vi "Obtain Notifier.vi"(7 "Notifier Name":string, 8 "error in":errorcluster, 10 "IMessagePayload.lvclass":refnum<class "IMessagePayload.lvclass">, 11 "NotifierMessageTransport in":refnum<class "NotifierMessageTransport.lvclass">) -> (0 "error out":errorcluster, 3 "NotifierMessageTransport out":refnum<class "NotifierMessageTransport.lvclass">)   [LabVIEW 2016, in "NotifierMessageTransport.lvclass"]
uses:
  NotifierMessageTransport.lvclass
  IMessagePayload/IMessagePayload.lvclass
  NotifierMessageTransport.lvclass/NotifierMessageTransport.ctl
panel:
  # "INPUTS"
  # "OUTPUTS"
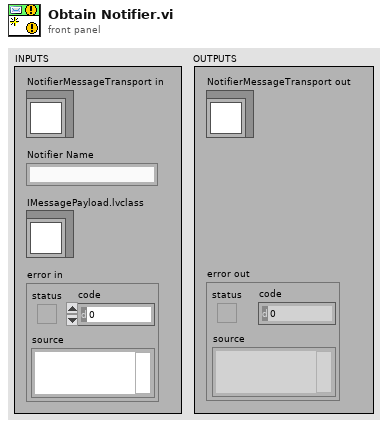
[diagram p1: front panel]
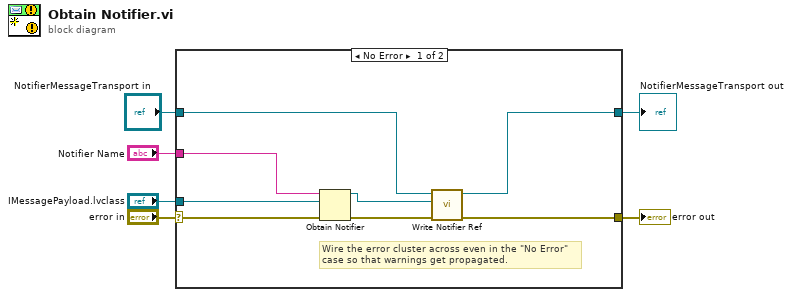
[diagram p0: block diagram]
diagram:
  n1 = case shown="No Error" "error in" {
    selector: "error in" -> [w14 w16]
    tunnel: [w7 w16] -> w5
    tunnel: [w8 w15] -> w3
    tunnel: "NotifierMessageTransport in" -> [w9 w15]
    tunnel: "IMessagePayload.lvclass" -> [w13 _]
    tunnel: "Notifier Name" -> [w12 _]
    frame No Error {
      # "Wire the error cluster across even in the \"No Error\"\ncase so that warnings get propagated."
      n2 = Obtain Notifier(name (unnamed)=w12, notification data type=w13, error in (no error)=w14) -> (notifier out=w10:refnum<notifier>, error out=w11:errorcluster)  [unwired: 1 in, 1 out]
      n3 = call "Write Notifier Ref.vi"("error in"=w11, "Notifier Ref"=w10, "NotifierMessageTransport in"=w9) -> ("error out"=w7:errorcluster, "NotifierMessageTransport out"=w8:refnum<class "NotifierMessageTransport.lvclass">)  [unwired: 7 in]
    }
    frame Error {
    }
  }
  "error out" <- w5
  "NotifierMessageTransport out" <- w3
